vi "PolarizationSimulation.vi"() -> ()   [LabVIEW 2018]
uses:
  <vilib>/Analysis/NI_AALPro.lvlib
  <vilib>/Analysis/NI_AALBase.lvlib
panel:
  in  "STOP":bool
  in  "Microwave Power":dbl=1.0
  in  "Lower Fit\nParameter":dbl=-3.6
  in  "Upper Fit\nParameter":dbl=3.6
  in  "Std Dev Noise":dbl=0.003 step=0.0001
  out "lower x-value":dbl
  out "upper x-value":dbl
  in  "RF Control":cluster{i32, i32}(slide)={200, 230} scale=0.0..500.0
  out "p":dbl
  out "r":dbl
  in  "Saturation\nPolarization":dbl=0.8 min=0.0 max=0.99 step=0.01
  out "Reimann \nsum of Q":dbl
  out "Corrected Data (Q)":cluster{dbl[], dbl[]}(graph)
  out "Population Graphs":cluster{dbl[], "Array out":dbl[]}[](graph)
  in  "Select Target Type":u16(ring)=2 items=["H Target", "Test Case", "Deuteron"]
  in  "Reset":bool
  out "Total Polarization (P)":cluster{dbl, dbl}(graph)
  in  "Spin Manipulation\nPower Factor":dbl=0.005
  in  "Decay Spin\nManipulation":bool
  out "Reimann\nsum of P":dbl
  out "Corrected Data (P)":cluster{dbl[], dbl[]}[](graph)
  out "Signal and Fit (P)":cluster{dbl[], "Best Polynomial Fit":dbl[]}[](graph)
  in  "Positive\nPolarization":bool
  in  "Microwave on":bool
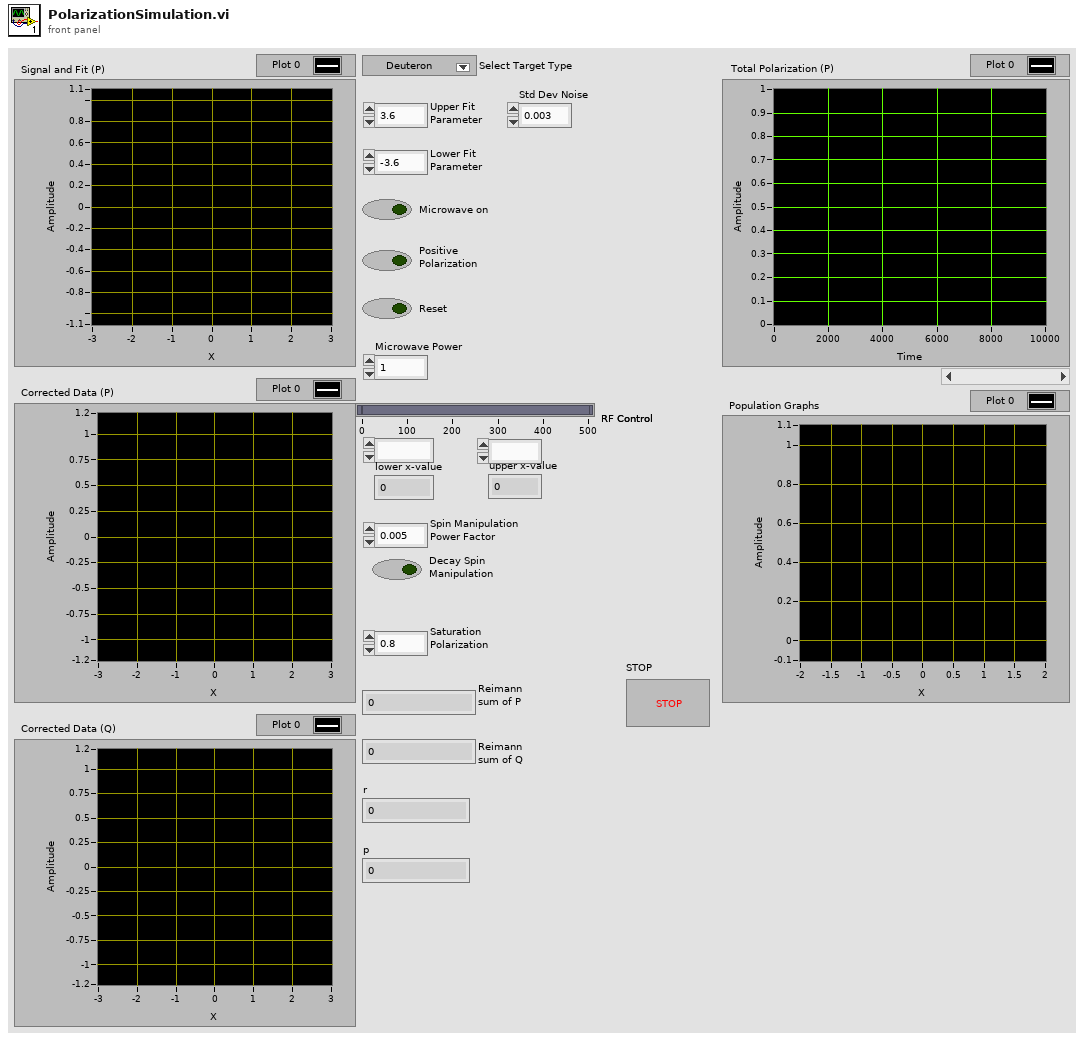
[diagram p1: front panel]
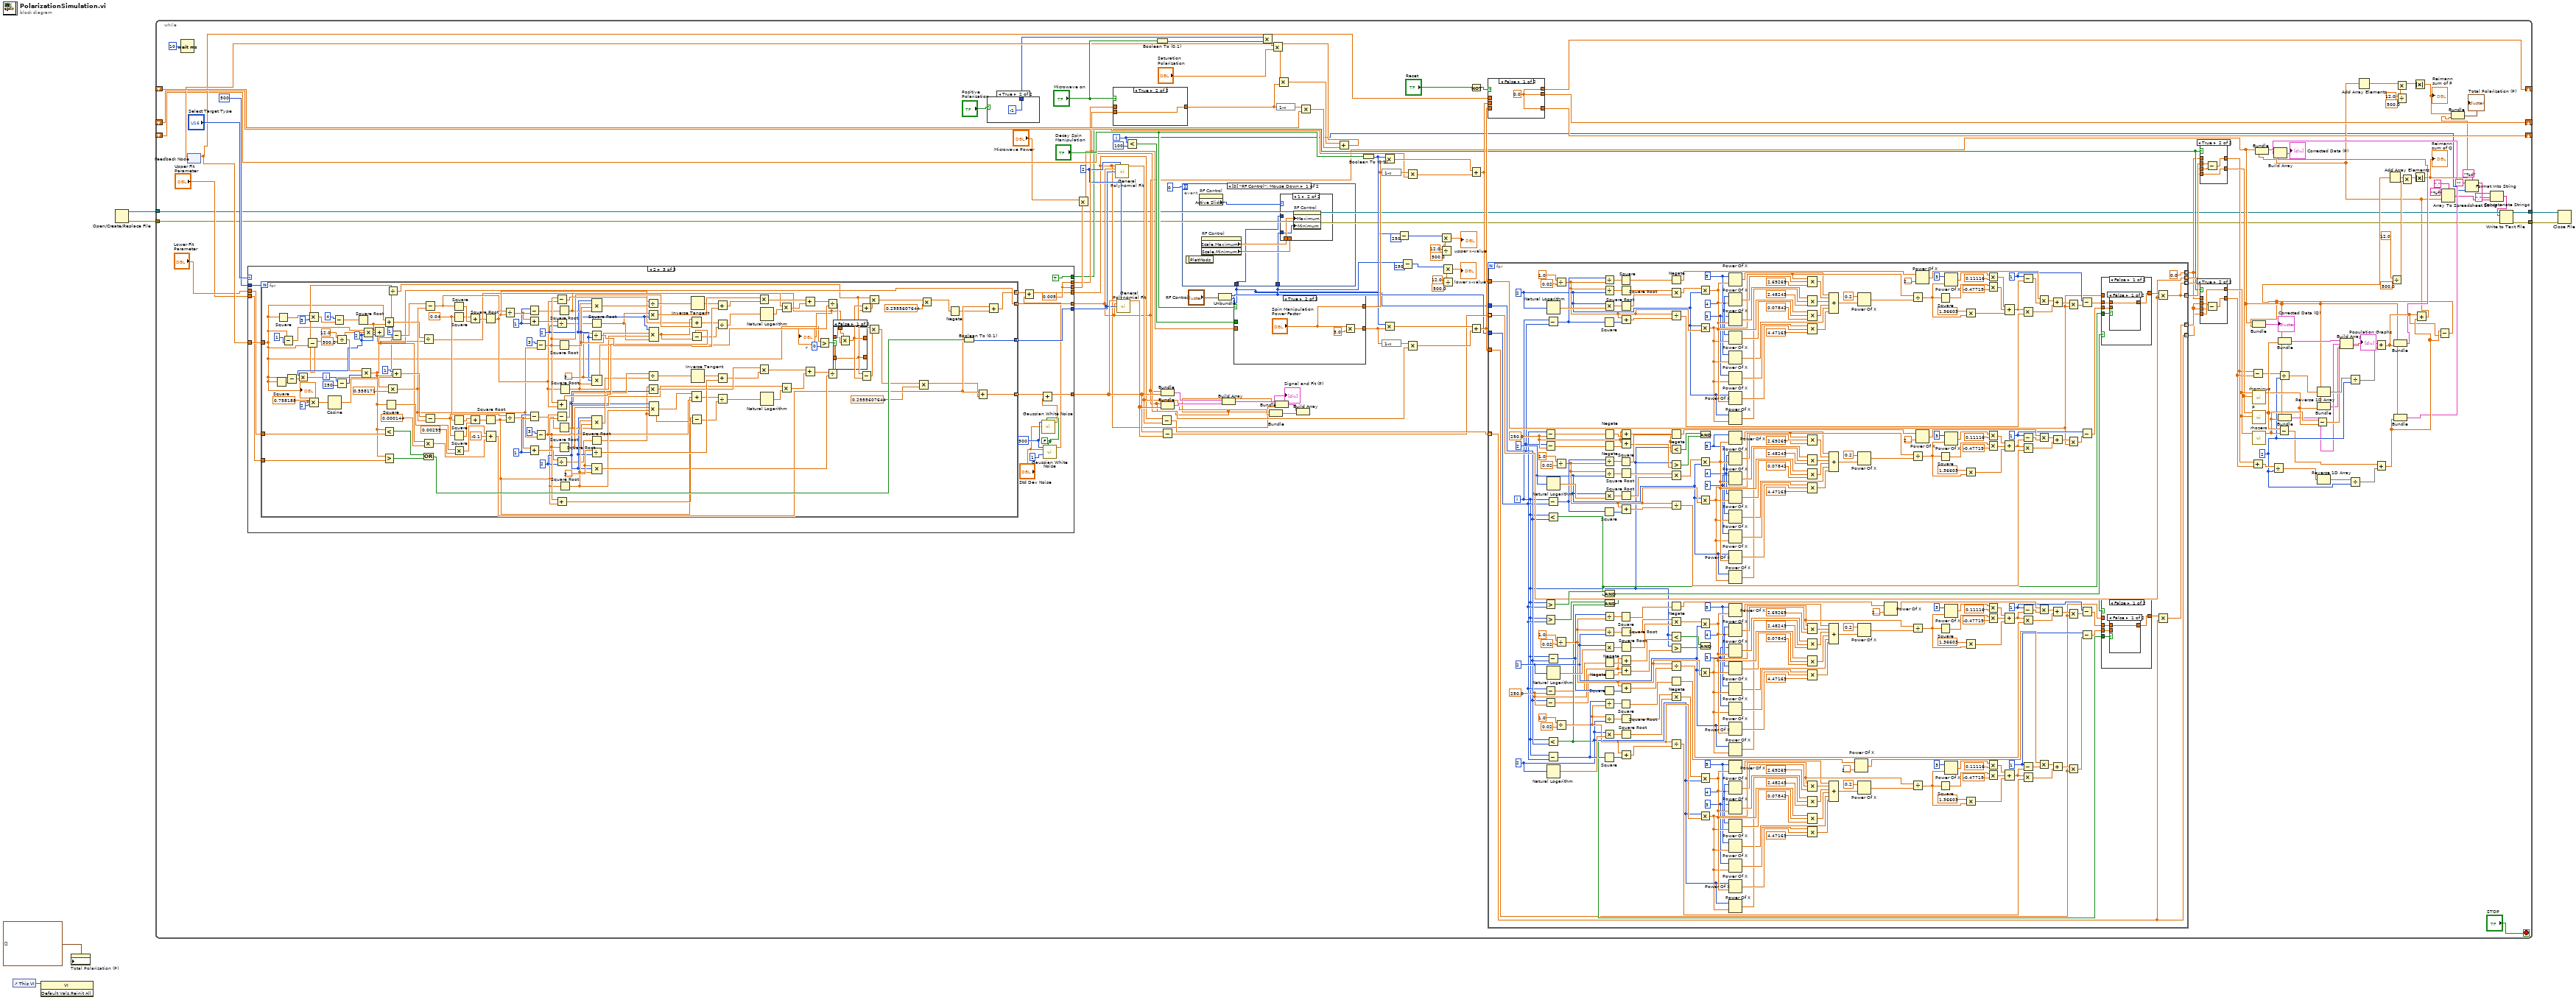
[diagram p0: block diagram]
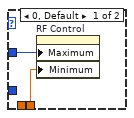
[diagram p2: hidden frame]
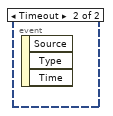
[diagram p3: hidden frame]
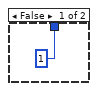
[diagram p4: hidden frame]
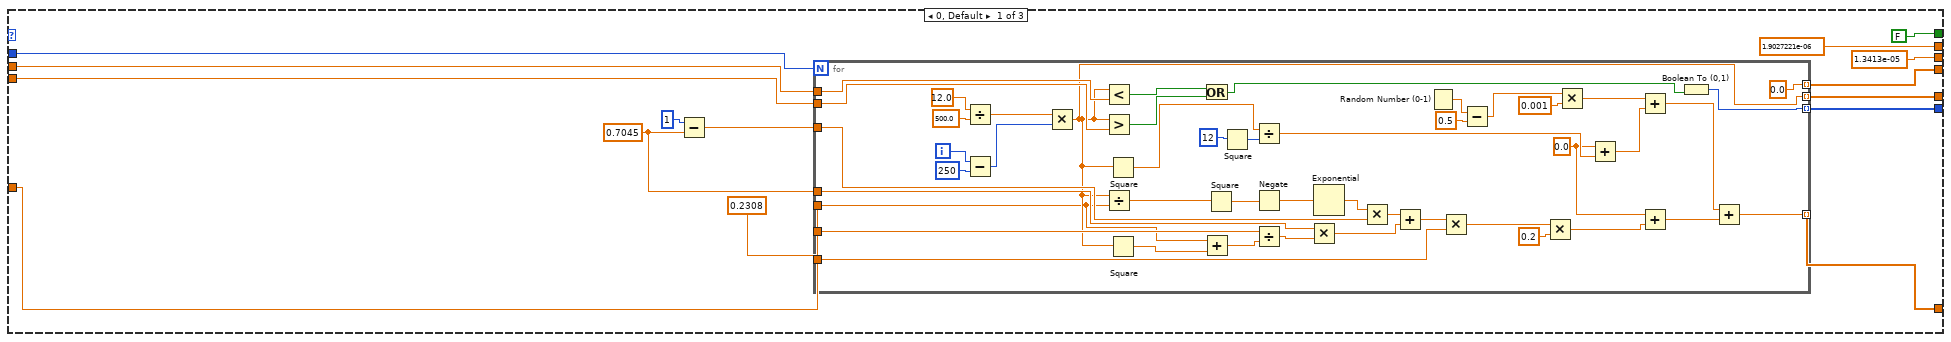
[diagram p5: hidden frame]
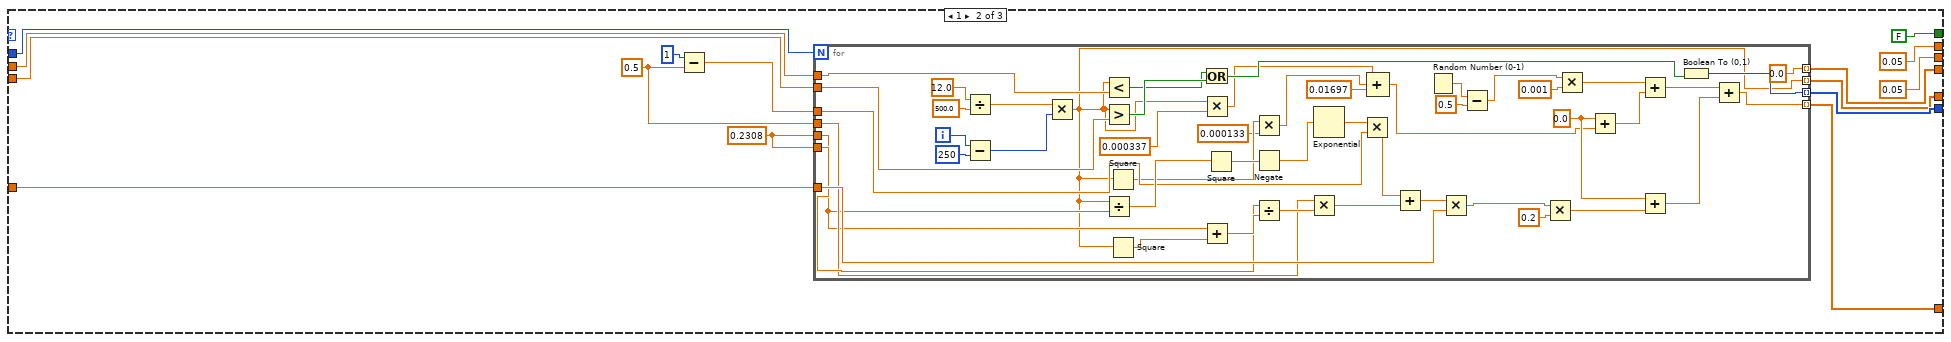
[diagram p6: hidden frame]
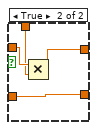
[diagram p7: hidden frame]
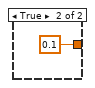
[diagram p9: hidden frame]
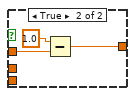
[diagram p15: hidden frame]
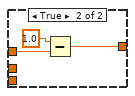
[diagram p17: hidden frame]
diagram:
  n1 = control-ref of="This VI"() -> (w6:refnum<vi>)
  n2 = invoke class="VI" method="Default Vals.Reinit All"(reference=w6) -> ()  [unwired: 2 in, 3 out]
  n3 = property on="Total Polarization (P)" class="WFChart (strict)"("History Data"=cluster{dbl, dbl}[] []) -> ()  [unwired: 2 in, 2 out]
  n4 = Open/Create/Replace File() -> (refnum out=w4:refnum<file>, error out=w3:errorcluster)  [unwired: 6 in, 1 out]
  n5 = while {
    shift-right: [w130] -> _
    shift-left: _ -> [w137]
    shift-right: [w129] -> _
    shift-left: _ -> [w109]
    shift-right: [w104] -> _
    shift-left: _ -> [w103]
    tunnel: w4 -> [w21]
    tunnel: w3 -> [w20]
    tunnel: [w19] -> w2
    tunnel: [w18] -> w1
    i -> [w13]
    stop <- "STOP" stop-if-true
    w83 = 2
    w115 = 2
    n6 = Wait (ms)(milliseconds to wait=10) -> ()  [unwired: 1 out]
    n7 = feedback #1() -> (w113:dbl)  [unwired: 1 in]
    n8 = case shown="2" "Select Target Type" {
      tunnel: [1.3413e-05 ("Growth Constant") 0.05 ("Growth Constant") w292] -> w121
      tunnel: [1.9027221e-06 ("Decay Constant") 0.05 ("Decay Constant") w292] -> w120
      tunnel: 500 -> [w167 w228 w296]
      tunnel: w113 -> [w166 w227 w299]
      tunnel: "Upper Fit\nParameter" -> [w165 w225 w297]
      tunnel: "Lower Fit\nParameter" -> [w164 w226 w298]
      tunnel: [w160 w223 w294] -> w60
      tunnel: [w163 w222 w288] -> w118
      tunnel: [w162 w224 w295] -> w114
      tunnel: [FALSE FALSE TRUE] -> w96
      tunnel: [w157 w218 w286] -> w59
      frame 0, Default {
        w158 = 0.2308
        w159 = 0.7045
        n9 = Subtract(x=1, y=w159) -> (x-y=w169:dbl)
        n10 = for {
          N: w167 -> [_]
          tunnel: w166 -> [w215]
          tunnel: [w177] -> w160 mode=indexing
          tunnel: [w193] -> w163 mode=indexing
          tunnel: [w208] -> w162 mode=indexing
          tunnel: w169 -> [w202]
          tunnel: w158 -> [w200]
          tunnel: w158 -> [w175]
          tunnel: w159 -> [w194]
          tunnel: w165 -> [w187]
          tunnel: w164 -> [w186]
          tunnel: [0.0] -> w157 mode=indexing
          i -> [w176]
          w192 = 0.0
          n11 = Divide(x=12.0, y=500.0) -> (x/y=w178:dbl)
          n12 = Subtract(x=w176, y=250) -> (x-y=w182:i32)
          n13 = Multiply(x=w178, y=w182) -> (x*y=w177:dbl)
          n14 = Less?(x=w177, y=w186) -> (x < y?=w204:bool)
          n15 = Greater?(x=w177, y=w187) -> (0:w205:bool)
          n16 = Divide(x=w177, y=w175) -> (x/y=w216:dbl)
          n17 = Square(x=w177) -> (x^2=w214:dbl)
          n18 = Square(x=w177) -> (x^2=w199:dbl)
          n19 = Or(x=w204, y=w205) -> (x .or. y?=w206:bool)
          n20 = Add(x=w175, y=w199) -> (x+y=w201:dbl)
          n21 = Square(x=w216) -> (x^2=w217:dbl)
          n22 = Square(x=12) -> (x^2=w213:i32)
          n23 = Divide(x=w214, y=w213) -> (x/y=w203:dbl)
          n24 = Negate(x=w217) -> (-x=w189:dbl)
          n25 = Divide(x=w200, y=w201) -> (x/y=w196:dbl)
          n26 = Multiply(x=w194, y=w196) -> (x*y=w195:dbl)
          n27 = Exponential(1:w189) -> (0:w188:dbl)
          n28 = Multiply(x=w188, y=w202) -> (x*y=w198:dbl)
          n29 = Add(x=w198, y=w195) -> (x+y=w197:dbl)
          n30 = Random Number (0-1)() -> (number: 0 to 1=w185:dbl)
          n31 = Multiply(x=w197, y=w215) -> (x*y=w211:dbl)
          n32 = Subtract(x=w185, y=0.5) -> (x-y=w184:dbl)
          n33 = Multiply(x=w211, y=0.2) -> (x*y=w174:dbl)
          n34 = Multiply(x=w184, y=0.001) -> (x*y=w209:dbl)
          n35 = Add(x=w192, y=w203) -> (x+y=w191:dbl)
          n36 = Add(x=w209, y=w191) -> (x+y=w207:dbl)
          n37 = Add(x=w192, y=w174) -> (x+y=w190:dbl)
          n38 = Boolean To (0,1)(Boolean=w206) -> (0, 1=w208:i16)
          n39 = Add(x=w207, y=w190) -> (x+y=w193:dbl)
        }
      }
      frame 1 {
        w229 = 0.2308
        w230 = 0.5
        n40 = Subtract(x=1, y=w230) -> (x-y=w232:dbl)
        n41 = for {
          N: w228 -> [_]
          tunnel: w227 -> [w279]
          tunnel: [w237] -> w223 mode=indexing
          tunnel: [w261] -> w222 mode=indexing
          tunnel: [w275] -> w224 mode=indexing
          tunnel: w232 -> [w270]
          tunnel: w229 -> [w268]
          tunnel: w229 -> [w244]
          tunnel: w230 -> [w262]
          tunnel: w225 -> [w255]
          tunnel: w226 -> [w254]
          tunnel: [0.0] -> w218 mode=indexing
          i -> [w245]
          w260 = 0.0
          n42 = Divide(x=12.0, y=500.0) -> (x/y=w246:dbl)
          n43 = Subtract(x=w245, y=250) -> (x-y=w250:i32)
          n44 = Multiply(x=w246, y=w250) -> (x*y=w237:dbl)
          n45 = Less?(x=w237, y=w254) -> (x < y?=w271:bool)
          n46 = Greater?(x=w237, y=w255) -> (0:w272:bool)
          n47 = Divide(x=w237, y=w244) -> (x/y=w280:dbl)
          n48 = Square(x=w237) -> (x^2=w240:dbl)
          n49 = Square(x=w237) -> (x^2=w267:dbl)
          n50 = Or(x=w271, y=w272) -> (x .or. y?=w273:bool)
          n51 = Multiply(x=w237, y=0.000337) -> (x*y=w239:dbl)
          n52 = Add(x=w244, y=w267) -> (x+y=w269:dbl)
          n53 = Square(x=w280) -> (x^2=w281:dbl)
          n54 = Multiply(x=w240, y=0.000133) -> (x*y=w238:dbl)
          n55 = Negate(x=w281) -> (-x=w257:dbl)
          n56 = Divide(x=w268, y=w269) -> (x/y=w264:dbl)
          n57 = Multiply(x=w262, y=w264) -> (x*y=w263:dbl)
          n58 = Exponential(1:w257) -> (0:w256:dbl)
          n59 = Multiply(x=w256, y=w270) -> (x*y=w266:dbl)
          n60 = Compound Arithmetic op=ADD(w239, w238, 0.01697) -> (w241:dbl)
          n61 = Add(x=w266, y=w263) -> (x+y=w265:dbl)
          n62 = Random Number (0-1)() -> (number: 0 to 1=w253:dbl)
          n63 = Multiply(x=w265, y=w279) -> (x*y=w278:dbl)
          n64 = Subtract(x=w253, y=0.5) -> (x-y=w252:dbl)
          n65 = Multiply(x=w278, y=0.2) -> (x*y=w243:dbl)
          n66 = Multiply(x=w252, y=0.001) -> (x*y=w276:dbl)
          n67 = Add(x=w260, y=w241) -> (x+y=w259:dbl)
          n68 = Add(x=w276, y=w259) -> (x+y=w274:dbl)
          n69 = Add(x=w260, y=w243) -> (x+y=w258:dbl)
          n70 = Boolean To (0,1)(Boolean=w273) -> (0, 1=w275:i16)
          n71 = Add(x=w274, y=w258) -> (x+y=w261:dbl)
        }
      }
      frame 2 {
        w283 = FALSE
        w289 = 500
        w292 = 0.005
        n72 = for {
          N: w296 -> [_]
          tunnel: [w332] -> w294 mode=indexing
          tunnel: [w421] -> w295 mode=indexing
          tunnel: w297 -> [w420]
          tunnel: w298 -> [w419]
          tunnel: [w323] -> w293 mode=indexing
          tunnel: w299 -> [w300]
          tunnel: [w324] -> w290 mode=indexing
          i -> [w397]
          w315 = 2
          w358 = 1
          w362 = 3.141592653589793
          w356 = 2
          w341 = 0.04
          w394 = 1
          w399 = 3.141592653589793
          w392 = 2
          n73 = Square(x=w300) -> (x^2=w318:dbl)
          n74 = Square(x=w300) -> (x^2=w348:dbl)
          n75 = Subtract(x=w300, y=1) -> (x-y=w343:dbl)
          n76 = Subtract(x=w300, y=w318) -> (x-y=w317:dbl)
          n77 = Multiply(x=w315, y=w317) -> (x*y=w313:dbl)
          n78 = Multiply(x=w348, y=3) -> (x*y=w347:dbl)
          n79 = Multiply(x=0.758188, y=2) -> (x*y=w336:dbl)
          n80 = Cosine(x=w336) -> (cos(x)=w339:dbl)
          n81 = Subtract(x=4, y=w347) -> (x-y=w345:dbl)
          n82 = Divide(x=12.0, y=500.0) -> (x/y=w435:dbl)
          n83 = Subtract(x=w397, y=250) -> (x-y=w434:i32)
          n84 = Square Root(x=w345) -> (sqrt(x)=w316:dbl)
          n85 = Multiply(x=w435, y=w434) -> (x*y=w332:dbl)
          n86 = Multiply(x=w343, y=w315) -> (x*y=w327:dbl)
          n87 = Add(x=w316, y=w315) -> (x+y=w314:dbl)
          n88 = Subtract(x=w314, y=w300) -> (x-y=w312:dbl)
          n89 = Add(x=w300, y=w316) -> (x+y=w344:dbl)
          n90 = Less?(x=w332, y=w419) -> (x < y?=w424:bool)
          n91 = Greater?(x=w332, y=w420) -> (0:w423:bool)
          n92 = Square(x=w332) -> (x^2=w334:dbl)
          n93 = Multiply(x=w339, y=0.558171) -> (x*y=w340:dbl)
          n94 = Divide(x=w313, y=w312) -> (x/y=w311:dbl)
          n95 = Subtract(x=1, y=w332) -> (x-y=w429:dbl)
          n96 = Add(x=1, y=w332) -> (x+y=w386:dbl)
          n97 = Divide(x=w344, y=w327) -> (x/y=w319:dbl)
          "r" <- w319
          n98 = Multiply(x=w332, y=0.000144) -> (x*y=w329:dbl)
          n99 = Or(x=w424, y=w423) -> (x .or. y?=w422:bool)
          n100 = Subtract(x=w429, y=w340) -> (x-y=w425:dbl)
          n101 = Subtract(x=w386, y=w340) -> (x-y=w382:dbl)
          n102 = Square(x=w425) -> (x^2=w428:dbl)
          n103 = Square(x=w341) -> (x^2=w427:dbl)
          n104 = Square(x=w341) -> (x^2=w384:dbl)
          n105 = Square(x=w382) -> (x^2=w385:dbl)
          n106 = Multiply(x=w334, y=0.00295) -> (x*y=w333:dbl)
          n107 = Add(x=w427, y=w428) -> (x+y=w426:dbl)
          n108 = Add(x=w384, y=w385) -> (x+y=w383:dbl)
          n109 = Square Root(x=w426) -> (sqrt(x)=w389:dbl)
          n110 = Square Root(x=w383) -> (sqrt(x)=w353:dbl)
          n111 = Compound Arithmetic op=ADD(w333, -0.1, w329) -> (w325:dbl)
          n112 = Divide(x=w425, y=w389) -> (x/y=w395:dbl)
          n113 = Divide(x=w382, y=w353) -> (x/y=w359:dbl)
          n114 = Subtract(x=w394, y=w395) -> (x-y=w350:dbl)
          n115 = Add(x=w395, y=w394) -> (x+y=w393:dbl)
          n116 = Subtract(x=w358, y=w359) -> (x-y=w351:dbl)
          n117 = Add(x=w359, y=w358) -> (x+y=w357:dbl)
          n118 = Subtract(x=3, y=w340) -> (x-y=w405:dbl)
          n119 = Subtract(x=3, y=w340) -> (x-y=w368:dbl)
          n120 = Subtract(x=w405, y=w389) -> (x-y=w414:dbl)
          n121 = Divide(x=w393, y=w392) -> (x/y=w391:dbl)
          n122 = Add(x=w405, y=w389) -> (x+y=w404:dbl)
          n123 = Subtract(x=w368, y=w353) -> (x-y=w377:dbl)
          n124 = Divide(x=w357, y=w356) -> (x/y=w355:dbl)
          n125 = Add(x=w368, y=w353) -> (x+y=w367:dbl)
          n126 = Square Root(x=w350) -> (sqrt(x)=w396:dbl)
          n127 = Square Root(x=w405) -> (sqrt(x)=w408:dbl)
          n128 = Square Root(x=w351) -> (sqrt(x)=w360:dbl)
          n129 = Square Root(x=w368) -> (sqrt(x)=w371:dbl)
          n130 = Square Root(x=w389) -> (sqrt(x)=w398:dbl)
          n131 = Square Root(x=w353) -> (sqrt(x)=w361:dbl)
          n132 = Square Root(x=w391) -> (sqrt(x)=w390:dbl)
          n133 = Divide(x=w399, y=w392) -> (x/y=w416:dbl)
          n134 = Square Root(x=w355) -> (sqrt(x)=w354:dbl)
          n135 = Divide(x=w362, y=w356) -> (x/y=w379:dbl)
          n136 = Compound Arithmetic op=MULTIPLY(w392, w398, w408, w396) -> (w413:dbl)
          n137 = Compound Arithmetic op=MULTIPLY(w399, w392, w398) -> (w400:dbl)
          n138 = Compound Arithmetic op=MULTIPLY(w356, w361, w371, w360) -> (w376:dbl)
          n139 = Compound Arithmetic op=MULTIPLY(w362, w356, w361) -> (w363:dbl)
          n140 = Divide(x=w414, y=w413) -> (x/y=w412:dbl)
          n141 = Multiply(x=w390, y=w392) -> (x*y=w418:dbl)
          n142 = Divide(x=w377, y=w376) -> (x/y=w375:dbl)
          n143 = Multiply(x=w354, y=w356) -> (x*y=w381:dbl)
          n144 = Compound Arithmetic op=MULTIPLY(w392, w408, w398, w390) -> (w403:dbl)
          n145 = Compound Arithmetic op=MULTIPLY(w356, w371, w361, w354) -> (w366:dbl)
          n146 = Subtract(x=w404, y=w403) -> (x-y=w402:dbl)
          n147 = Subtract(x=w367, y=w366) -> (x-y=w365:dbl)
          n148 = Inverse Tangent(1:w412) -> (0:w417:dbl)
          n149 = Inverse Tangent(1:w375) -> (0:w380:dbl)
          n150 = Compound Arithmetic op=ADD(w403, w389, w405) -> (w407:dbl)
          n151 = Compound Arithmetic op=ADD(w366, w353, w368) -> (w370:dbl)
          n152 = Add(x=w417, y=w416) -> (x+y=w415:dbl)
          n153 = Divide(x=w407, y=w402) -> (x/y=w406:dbl)
          n154 = Add(x=w380, y=w379) -> (x+y=w378:dbl)
          n155 = Divide(x=w370, y=w365) -> (x/y=w369:dbl)
          n156 = Multiply(x=w418, y=w415) -> (x*y=w411:dbl)
          n157 = Multiply(x=w381, y=w378) -> (x*y=w374:dbl)
          n158 = Natural Logarithm(1:w406) -> (0:w409:dbl)
          n159 = Natural Logarithm(1:w369) -> (0:w372:dbl)
          n160 = Multiply(x=w396, y=w409) -> (x*y=w410:dbl)
          n161 = Multiply(x=w360, y=w372) -> (x*y=w373:dbl)
          n162 = Add(x=w411, y=w410) -> (x+y=w401:dbl)
          n163 = Add(x=w374, y=w373) -> (x+y=w364:dbl)
          n164 = Greater?(x=w300, y=0) -> (0:w302:bool)
          n165 = Divide(x=w401, y=w400) -> (x/y=w342:dbl)
          n166 = Divide(x=w364, y=w363) -> (x/y=w304:dbl)
          n167 = case shown="False" w302 {
            tunnel: w342 -> [w439 w444]
            tunnel: [w437 w443] -> w322
            tunnel: w319 -> [w440 w442]
            tunnel: w304 -> [w438 w441]
            tunnel: [w438 w441] -> w303
            frame False {
              n168 = Multiply(x=w440, y=w439) -> (x*y=w437:dbl)
            }
            frame True {
              n169 = Multiply(x=w444, y=w442) -> (x*y=w443:dbl)
            }
          }
          n170 = Add(x=w322, y=w303) -> (x+y=w326:dbl)
          n171 = Subtract(x=w303, y=w322) -> (x-y=w352:dbl)
          n172 = Multiply(x=w311, y=w326) -> (x*y=w310:dbl)
          n173 = Multiply(x=w311, y=w352) -> (x*y=w309:dbl)
          n174 = Multiply(x=w309, y=0.2955607644) -> (x*y=w306:dbl)
          n175 = Multiply(x=w310, y=0.2955607644) -> (x*y=w308:dbl)
          n176 = Negate(x=w308) -> (-x=w321:dbl)
          n177 = Boolean To (0,1)(Boolean=w422) -> (0, 1=w421:i16)
          n178 = Add(x=w325, y=w306) -> (x+y=w323:dbl)
          n179 = Add(x=w325, y=w321) -> (x+y=w324:dbl)
          "p" <- w300
        }
        n180 = call <vilib>:"Gaussian White Noise.vi"("initialize?"=w283, "standard deviation"="Std Dev Noise", "samples"=w289) -> ("Gaussian noise pattern"=w287:dbl[])  [unwired: 7 in, 1 out]
        n181 = Add(x=w293, y=w287) -> (x+y=w288:dbl[])
        n182 = call <vilib>:"Gaussian White Noise.vi"("initialize?"=w283, "seed"=1, "standard deviation"="Std Dev Noise", "samples"=w289) -> ("Gaussian noise pattern"=w285:dbl[])  [unwired: 6 in, 1 out]
        n183 = Add(x=w290, y=w285) -> (x+y=w286:dbl[])
      }
    }
    n184 = case shown="True" "Positive\nPolarization" {
      tunnel: [1 -1] -> w56
      frame False {
      }
      frame True {
      }
    }
    n185 = Multiply(x="Microwave Power", y=w121) -> (x*y=w24:dbl)
    n186 = case shown="True" "Microwave on" {
      tunnel: [w453 w454] -> w124
      tunnel: w24 -> [_ w454]
      tunnel: w120 -> [w453 _]
      frame False {
      }
      frame True {
      }
    }
    n187 = call <vilib>:"General Polynomial Fit.vi"("Y"=w59, "polynomial order"=w115, "X"=w60, "Weight"=w114) -> ("Best Polynomial Fit"=w62:dbl[])  [unwired: 8 in, 3 out]
    n188 = call <vilib>:"General Polynomial Fit.vi"("Y"=w118, "polynomial order"=w115, "X"=w60, "Weight"=w114) -> ("Best Polynomial Fit"=w143:dbl[])  [unwired: 8 in, 3 out]
    n189 = Less?(x=w13, y=100) -> (x < y?=w132:bool)
    n190 = Boolean To (0,1)(Boolean="Microwave on") -> (0, 1=w139:i16)
    n191 = Subtract(x=w59, y=w62) -> (x-y=w76:dbl[])
    n192 = Bundle(w60, w118) -> (w144:cluster{dbl[], dbl[]})  [unwired: 1 in]
    n193 = Bundle(w60, "Best Polynomial Fit"=w143) -> (w64:cluster{dbl[], "Best Polynomial Fit":dbl[]})  [unwired: 1 in]
    n194 = Subtract(x=w118, y=w143) -> (x-y=w75:dbl[])
    n195 = Unbundle("RF Control") -> (w27:i32, w26:i32)
    n196 = event shown="[0] \"RF Control\": Mouse Down" {
      selector: _ -> [_ _]
      dyn-events: _ -> [_ _]
      timeout: 0 -> [_ _]
      tunnel: w27 -> [w147 _]
      tunnel: w26 -> [w146 _]
      event "RF Control": Mouse Down {
        n197 = event-data() -> ()  [unwired: 1 in, 1 out]
        n198 = property on="RF Control" class="Slide (strict)"() -> ("Active Slider"=w150:i32)  [unwired: 2 in, 2 out]
        n199 = property on="RF Control" class="Slide (strict)"() -> ("Scale.Maximum"=w148:dbl, "Scale.Minimum"=w149:dbl)  [unwired: 2 in, 2 out]
        n200 = case shown="1" w150 {
          tunnel: w149 -> [w152 _]
          tunnel: w146 -> [w151 _]
          tunnel: w148 -> [_ w154]
          tunnel: w147 -> [_ w153]
          frame 0, Default {
            n201 = property on="RF Control" class="Slide (strict)"("Maximum"=w151, "Minimum"=w152) -> ()  [unwired: 2 in, 2 out]
          }
          frame 1 {
            n202 = property on="RF Control" class="Slide (strict)"("Maximum"=w154, "Minimum"=w153) -> ()  [unwired: 2 in, 2 out]
          }
        }
      }
      event Timeout {
        n203 = event-data() -> ()  [unwired: 1 in, 3 out]
      }
    }
    n204 = Build Array(w144, w64) -> (→"Signal and Fit (P)":cluster{dbl[], "Best Polynomial Fit":dbl[]}[])
    n205 = case shown="True" "Decay Spin\nManipulation" {
      tunnel: [w445 "Spin Manipulation\nPower Factor"] -> w133
      tunnel: w24 -> [w447 _]
      tunnel: w132 -> [w446 _]
      tunnel: [w445 w450] -> w111
      frame False {
        n206 = case shown="False" w446 {
          tunnel: [w448 0.1] -> w445
          tunnel: w447 -> [w448 _]
          frame False {
          }
          frame True {
          }
        }
      }
      frame True {
        n207 = Multiply(x="Spin Manipulation\nPower Factor", y=3.0) -> (x*y=w450:dbl)
      }
    }
    n208 = Multiply(x=w56, y=w139) -> (x*y=w57:i32)
    n209 = Bundle(w60, "Best Polynomial Fit"=w62) -> (w63:cluster{dbl[], "Best Polynomial Fit":dbl[]})  [unwired: 1 in]
    n210 = Multiply(x=w57, y="Saturation\nPolarization") -> (x*y=w74:dbl)
    n211 = Bundle(w60, w59) -> (w61:cluster{dbl[], dbl[]})  [unwired: 1 in]
    n212 = expression code="1-x"(w124) -> (w140:dbl)
    n213 = Multiply(x=w74, y=w124) -> (x*y=w141:dbl)
    n214 = Build Array(w61, w63) -> ()  [unwired: 1 out]
    n215 = Multiply(x=w140, y=w137) -> (x*y=w142:dbl)
    n216 = Add(x=w141, y=w142) -> (x+y=w119:dbl)
    n217 = feedback-in #1(w119) -> ()
    n218 = Boolean To (0,1)(Boolean="Decay Spin\nManipulation") -> (0, 1=w112:i16)
    n219 = expression code="1-x"(w133) -> (w134:dbl)
    n220 = expression code="1-x"(w111) -> (w110:dbl)
    n221 = Multiply(x=w112, y=w133) -> (x*y=w135:dbl)
    n222 = Multiply(x=w112, y=w111) -> (x*y=w107:dbl)
    n223 = Subtract(x=w26, y=250) -> (x-y=w36:i32)
    n224 = Subtract(x=w27, y=250) -> (x-y=w33:i32)
    n225 = Multiply(x=w134, y=w109) -> (x*y=w136:dbl)
    n226 = Multiply(x=w110, y=w103) -> (x*y=w108:dbl)
    n227 = Divide(x=12.0, y=500.0) -> (x/y=w44:dbl)
    n228 = Multiply(x=w36, y=w44) -> (x*y=→"upper x-value":dbl)
    n229 = Divide(x=12.0, y=500.0) -> (x/y=w40:dbl)
    n230 = Multiply(x=w33, y=w40) -> (x*y=→"lower x-value":dbl)
    n231 = Not(x="Reset") -> (.not. x?=w127:bool)
    n232 = Add(x=w135, y=w136) -> (x+y=w128:dbl)
    n233 = Add(x=w107, y=w108) -> (x+y=w105:dbl)
    n234 = case shown="False" w127 {
      tunnel: [w467 w470] -> w130
      tunnel: w113 -> [_ w470]
      tunnel: [w467 w469] -> w129
      tunnel: w128 -> [_ w469]
      tunnel: w105 -> [_ w468]
      tunnel: [w467 w468] -> w104
      frame False {
        w467 = 0.0
      }
      frame True {
      }
    }
    n235 = for {
      tunnel: w75 -> [w614] mode=indexing
      tunnel: w128 -> [w622]
      tunnel: w26 -> [w478]
      tunnel: w27 -> [w477]
      tunnel: [w614] -> w117 mode=indexing
      tunnel: [w613] -> w106 mode=indexing
      tunnel: [w613] -> w116 mode=indexing
      tunnel: w76 -> [w472] mode=indexing
      tunnel: w105 -> [w476]
      tunnel: [w474] -> w101 mode=indexing
      tunnel: [w472] -> w100 mode=indexing
      tunnel: [0.0] -> w90 mode=indexing
      i -> [w475]
      w480 = 250.0
      w519 = 5
      w517 = 4
      w516 = 3
      w497 = 1
      w498 = 2
      w580 = 5
      w578 = 4
      w577 = 3
      w557 = 1
      w558 = 2
      w616 = 250.0
      w657 = 5
      w655 = 4
      w654 = 3
      w635 = 1
      w636 = 2
      w718 = 5
      w716 = 4
      w715 = 3
      w695 = 1
      w696 = 2
      n236 = Subtract(x=w477, y=w616) -> (x-y=w620:dbl)
      n237 = Subtract(x=w478, y=w616) -> (x-y=w621:dbl)
      n238 = Greater?(x=w475, y=w477) -> (0:w691:bool)
      n239 = Greater?(x=w475, y=w477) -> (0:w553:bool)
      n240 = Subtract(x=w477, y=w480) -> (x-y=w484:dbl)
      n241 = Subtract(x=w478, y=w480) -> (x-y=w485:dbl)
      n242 = Natural Logarithm(1:w636) -> (0:w670:dbl)
      n243 = Subtract(x=w475, y=w478) -> (x-y=w643:i32)
      n244 = Natural Logarithm(1:w696) -> (0:w731:dbl)
      n245 = Subtract(x=w475, y=w477) -> (x-y=w704:i32)
      n246 = Less?(x=w475, y=w478) -> (x < y?=w627:bool)
      n247 = Subtract(x=w475, y=w478) -> (x-y=w505:i32)
      n248 = Natural Logarithm(1:w498) -> (0:w532:dbl)
      n249 = Less?(x=w475, y=w478) -> (x < y?=w490:bool)
      n250 = Subtract(x=w475, y=w477) -> (x-y=w566:i32)
      n251 = Natural Logarithm(1:w558) -> (0:w593:dbl)
      n252 = Divide(x=1.0, y=0.02) -> (x/y=w640:dbl)
      n253 = Divide(x=1.0, y=0.02) -> (x/y=w700:dbl)
      n254 = Divide(x=1.0, y=0.02) -> (x/y=w502:dbl)
      n255 = Divide(x=1.0, y=0.02) -> (x/y=w562:dbl)
      n256 = Square(x=w643) -> (x^2=w644:i32)
      n257 = Square(x=w704) -> (x^2=w705:i32)
      n258 = Square(x=w505) -> (x^2=w506:i32)
      n259 = Square(x=w566) -> (x^2=w567:i32)
      n260 = Divide(x=w643, y=w640) -> (x/y=w647:dbl)
      n261 = Divide(x=w640, y=w636) -> (x/y=w668:dbl)
      n262 = Multiply(x=w636, y=w670) -> (x*y=w671:dbl)
      n263 = Negate(x=w620) -> (-x=w619:dbl)
      n264 = Negate(x=w621) -> (-x=w617:dbl)
      n265 = Divide(x=w704, y=w700) -> (x/y=w708:dbl)
      n266 = Divide(x=w700, y=w696) -> (x/y=w729:dbl)
      n267 = Multiply(x=w696, y=w731) -> (x*y=w732:dbl)
      n268 = Divide(x=w505, y=w502) -> (x/y=w509:dbl)
      n269 = Divide(x=w502, y=w498) -> (x/y=w530:dbl)
      n270 = Multiply(x=w498, y=w532) -> (x*y=w533:dbl)
      n271 = Negate(x=w484) -> (-x=w483:dbl)
      n272 = Negate(x=w485) -> (-x=w481:dbl)
      n273 = Divide(x=w566, y=w562) -> (x/y=w570:dbl)
      n274 = Divide(x=w562, y=w558) -> (x/y=w591:dbl)
      n275 = Multiply(x=w558, y=w593) -> (x*y=w594:dbl)
      n276 = And(x=w691, y=w627) -> (x .and. y?=w629:bool)
      n277 = And(x=w553, y=w490) -> (x .and. y?=w491:bool)
      n278 = Square(x=w647) -> (x^2=w649:dbl)
      n279 = Square(x=w708) -> (x^2=w710:dbl)
      n280 = Square(x=w509) -> (x^2=w511:dbl)
      n281 = Square(x=w570) -> (x^2=w572:dbl)
      n282 = Square Root(x=w668) -> (sqrt(x)=w669:dbl)
      n283 = Square Root(x=w671) -> (sqrt(x)=w672:dbl)
      n284 = Add(x=w640, y=w644) -> (x+y=w645:dbl)
      n285 = Add(x=w616, y=w619) -> (x+y=w618:dbl)
      n286 = Add(x=w616, y=w617) -> (x+y=w615:dbl)
      n287 = Square Root(x=w729) -> (sqrt(x)=w730:dbl)
      n288 = Square Root(x=w732) -> (sqrt(x)=w733:dbl)
      n289 = Add(x=w700, y=w705) -> (x+y=w706:dbl)
      n290 = Square Root(x=w530) -> (sqrt(x)=w531:dbl)
      n291 = Square Root(x=w533) -> (sqrt(x)=w534:dbl)
      n292 = Add(x=w480, y=w483) -> (x+y=w482:dbl)
      n293 = Add(x=w480, y=w481) -> (x+y=w479:dbl)
      n294 = Add(x=w502, y=w506) -> (x+y=w507:dbl)
      n295 = Square Root(x=w591) -> (sqrt(x)=w592:dbl)
      n296 = Square Root(x=w594) -> (sqrt(x)=w595:dbl)
      n297 = Add(x=w562, y=w567) -> (x+y=w568:dbl)
      n298 = Negate(x=w649) -> (-x=w648:dbl)
      n299 = Multiply(x=w669, y=w672) -> (x*y=w663:dbl)
      n300 = Divide(x=w640, y=w645) -> (x/y=w630:dbl)
      n301 = Negate(x=w710) -> (-x=w709:dbl)
      n302 = Less?(x=w475, y=w618) -> (x < y?=w624:bool)
      n303 = Greater?(x=w475, y=w615) -> (0:w623:bool)
      n304 = Multiply(x=w730, y=w733) -> (x*y=w724:dbl)
      n305 = Divide(x=w700, y=w706) -> (x/y=w703:dbl)
      n306 = Negate(x=w511) -> (-x=w510:dbl)
      n307 = Multiply(x=w531, y=w534) -> (x*y=w525:dbl)
      n308 = Less?(x=w475, y=w482) -> (x < y?=w487:bool)
      n309 = Greater?(x=w475, y=w479) -> (0:w486:bool)
      n310 = Divide(x=w502, y=w507) -> (x/y=w492:dbl)
      n311 = Negate(x=w572) -> (-x=w571:dbl)
      n312 = Multiply(x=w592, y=w595) -> (x*y=w586:dbl)
      n313 = Divide(x=w562, y=w568) -> (x/y=w565:dbl)
      n314 = Multiply(x=w663, y=w636) -> (x*y=w687:dbl)
      n315 = Multiply(x=w636, y=w640) -> (x*y=w681:dbl)
      n316 = Multiply(x=w724, y=w696) -> (x*y=w748:dbl)
      n317 = Multiply(x=w696, y=w700) -> (x*y=w742:dbl)
      n318 = Multiply(x=w525, y=w498) -> (x*y=w549:dbl)
      n319 = Multiply(x=w498, y=w502) -> (x*y=w543:dbl)
      n320 = Multiply(x=w586, y=w558) -> (x*y=w610:dbl)
      n321 = Multiply(x=w558, y=w562) -> (x*y=w604:dbl)
      n322 = And(x=w624, y=w623) -> ()  [unwired: 1 out]
      n323 = And(x=w487, y=w486) -> ()  [unwired: 1 out]
      n324 = Power Of X(1:w687, 2:w657) -> (0:w674:dbl)
      n325 = Power Of X(1:w687, 2:w655) -> (0:w680:dbl)
      n326 = Power Of X(1:w687, 2:w654) -> (0:w682:dbl)
      n327 = Power Of X(1:w681, 2:w655) -> (0:w686:dbl)
      n328 = Power Of X(1:w681, 2:w657) -> (0:w675:dbl)
      n329 = Power Of X(1:w681, 2:w654) -> (0:w684:dbl)
      n330 = Power Of X(1:w687, 2:w636) -> (0:w685:dbl)
      n331 = Power Of X(1:w681, 2:w636) -> (0:w683:dbl)
      n332 = Power Of X(1:w748, 2:w718) -> (0:w735:dbl)
      n333 = Power Of X(1:w748, 2:w716) -> (0:w741:dbl)
      n334 = Power Of X(1:w748, 2:w715) -> (0:w743:dbl)
      n335 = Power Of X(1:w742, 2:w716) -> (0:w747:dbl)
      n336 = Power Of X(1:w742, 2:w718) -> (0:w736:dbl)
      n337 = Power Of X(1:w742, 2:w715) -> (0:w745:dbl)
      n338 = Power Of X(1:w748, 2:w696) -> (0:w746:dbl)
      n339 = Power Of X(1:w742, 2:w696) -> (0:w744:dbl)
      n340 = Power Of X(1:w549, 2:w519) -> (0:w536:dbl)
      n341 = Power Of X(1:w549, 2:w517) -> (0:w542:dbl)
      n342 = Power Of X(1:w549, 2:w516) -> (0:w544:dbl)
      n343 = Power Of X(1:w543, 2:w517) -> (0:w548:dbl)
      n344 = Power Of X(1:w543, 2:w519) -> (0:w537:dbl)
      n345 = Power Of X(1:w543, 2:w516) -> (0:w546:dbl)
      n346 = Power Of X(1:w549, 2:w498) -> (0:w547:dbl)
      n347 = Power Of X(1:w543, 2:w498) -> (0:w545:dbl)
      n348 = Power Of X(1:w610, 2:w580) -> (0:w597:dbl)
      n349 = Power Of X(1:w610, 2:w578) -> (0:w603:dbl)
      n350 = Power Of X(1:w610, 2:w577) -> (0:w605:dbl)
      n351 = Power Of X(1:w604, 2:w578) -> (0:w609:dbl)
      n352 = Power Of X(1:w604, 2:w580) -> (0:w598:dbl)
      n353 = Power Of X(1:w604, 2:w577) -> (0:w607:dbl)
      n354 = Power Of X(1:w610, 2:w558) -> (0:w608:dbl)
      n355 = Power Of X(1:w604, 2:w558) -> (0:w606:dbl)
      n356 = Compound Arithmetic op=MULTIPLY(w681, w680, 2.69269) -> (w676:dbl)
      n357 = Compound Arithmetic op=MULTIPLY(w682, w683, 2.48243) -> (w678:dbl)
      n358 = Compound Arithmetic op=MULTIPLY(w687, w686, 0.07842) -> (w677:dbl)
      n359 = Compound Arithmetic op=MULTIPLY(w684, w685, 4.47163) -> (w679:dbl)
      n360 = Compound Arithmetic op=MULTIPLY(w742, w741, 2.69269) -> (w737:dbl)
      n361 = Compound Arithmetic op=MULTIPLY(w743, w744, 2.48243) -> (w739:dbl)
      n362 = Compound Arithmetic op=MULTIPLY(w748, w747, 0.07842) -> (w738:dbl)
      n363 = Compound Arithmetic op=MULTIPLY(w745, w746, 4.47163) -> (w740:dbl)
      n364 = Compound Arithmetic op=MULTIPLY(w543, w542, 2.69269) -> (w538:dbl)
      n365 = Compound Arithmetic op=MULTIPLY(w544, w545, 2.48243) -> (w540:dbl)
      n366 = Compound Arithmetic op=MULTIPLY(w549, w548, 0.07842) -> (w539:dbl)
      n367 = Compound Arithmetic op=MULTIPLY(w546, w547, 4.47163) -> (w541:dbl)
      n368 = Compound Arithmetic op=MULTIPLY(w604, w603, 2.69269) -> (w599:dbl)
      n369 = Compound Arithmetic op=MULTIPLY(w605, w606, 2.48243) -> (w601:dbl)
      n370 = Compound Arithmetic op=MULTIPLY(w610, w609, 0.07842) -> (w600:dbl)
      n371 = Compound Arithmetic op=MULTIPLY(w607, w608, 4.47163) -> (w602:dbl)
      n372 = Compound Arithmetic op=unknown(w674, w676, w678, w677, w675, w679) -> (w637:dbl)
      n373 = Compound Arithmetic op=unknown(w735, w737, w739, w738, w736, w740) -> (w697:dbl)
      n374 = Compound Arithmetic op=unknown(w536, w538, w540, w539, w537, w541) -> (w499:dbl)
      n375 = Compound Arithmetic op=unknown(w597, w599, w601, w600, w598, w602) -> (w559:dbl)
      n376 = Power Of X(1:2.718281828459045, 2:w571) -> (0:w569:dbl)
      n377 = Power Of X(1:w637, 2:0.2) -> (0:w689:dbl)
      n378 = Power Of X(1:w697, 2:0.2) -> (0:w750:dbl)
      n379 = Power Of X(1:w499, 2:0.2) -> (0:w551:dbl)
      n380 = Power Of X(1:w559, 2:0.2) -> (0:w612:dbl)
      n381 = Power Of X(1:2.718281828459045, 2:w510) -> (0:w508:dbl)
      n382 = Divide(x=w681, y=w689) -> (x/y=w673:dbl)
      n383 = Divide(x=w742, y=w750) -> (x/y=w734:dbl)
      n384 = Divide(x=w543, y=w551) -> (x/y=w535:dbl)
      n385 = Divide(x=w604, y=w612) -> (x/y=w596:dbl)
      n386 = Power Of X(1:2.718281828459045, 2:w648) -> (0:w646:dbl)
      n387 = Power Of X(1:2.718281828459045, 2:w709) -> (0:w707:dbl)
      n388 = Square(x=w673) -> (x^2=w667:dbl)
      n389 = Square(x=w734) -> (x^2=w728:dbl)
      n390 = Square(x=w535) -> (x^2=w529:dbl)
      n391 = Square(x=w596) -> (x^2=w590:dbl)
      n392 = Power Of X(1:w673, 2:3) -> (0:w666:dbl)
      n393 = Power Of X(1:w734, 2:3) -> (0:w727:dbl)
      n394 = Power Of X(1:w535, 2:3) -> (0:w528:dbl)
      n395 = Power Of X(1:w596, 2:3) -> (0:w589:dbl)
      n396 = Multiply(x=1.36603, y=w673) -> (x*y=w688:dbl)
      n397 = Multiply(x=1.36603, y=w734) -> (x*y=w749:dbl)
      n398 = Multiply(x=1.36603, y=w535) -> (x*y=w550:dbl)
      n399 = Multiply(x=1.36603, y=w596) -> (x*y=w611:dbl)
      n400 = Multiply(x=w666, y=0.11116) -> (x*y=w665:dbl)
      n401 = Multiply(x=w667, y=-0.47719) -> (x*y=w664:dbl)
      n402 = Multiply(x=w727, y=0.11116) -> (x*y=w726:dbl)
      n403 = Multiply(x=w728, y=-0.47719) -> (x*y=w725:dbl)
      n404 = Multiply(x=w528, y=0.11116) -> (x*y=w527:dbl)
      n405 = Multiply(x=w529, y=-0.47719) -> (x*y=w526:dbl)
      n406 = Multiply(x=w589, y=0.11116) -> (x*y=w588:dbl)
      n407 = Multiply(x=w590, y=-0.47719) -> (x*y=w587:dbl)
      n408 = Compound Arithmetic op=unknown(w665, w664, w688) -> (w641:dbl)
      n409 = Compound Arithmetic op=unknown(w726, w725, w749) -> (w701:dbl)
      n410 = Compound Arithmetic op=unknown(w527, w526, w550) -> (w503:dbl)
      n411 = Compound Arithmetic op=unknown(w588, w587, w611) -> (w563:dbl)
      n412 = Subtract(x=w635, y=w641) -> (x-y=w638:dbl)
      n413 = Multiply(x=w641, y=w630) -> (x*y=w642:dbl)
      n414 = Subtract(x=w695, y=w701) -> (x-y=w698:dbl)
      n415 = Multiply(x=w701, y=w703) -> (x*y=w702:dbl)
      n416 = Subtract(x=w497, y=w503) -> (x-y=w500:dbl)
      n417 = Multiply(x=w503, y=w492) -> (x*y=w504:dbl)
      n418 = Subtract(x=w557, y=w563) -> (x-y=w560:dbl)
      n419 = Multiply(x=w563, y=w565) -> (x*y=w564:dbl)
      n420 = Multiply(x=w646, y=w638) -> (x*y=w639:dbl)
      n421 = Multiply(x=w707, y=w698) -> (x*y=w699:dbl)
      n422 = Multiply(x=w508, y=w500) -> (x*y=w501:dbl)
      n423 = Multiply(x=w569, y=w560) -> (x*y=w561:dbl)
      n424 = Add(x=w639, y=w642) -> (x+y=w634:dbl)
      n425 = Add(x=w699, y=w702) -> (x+y=w694:dbl)
      n426 = Add(x=w501, y=w504) -> (x+y=w496:dbl)
      n427 = Add(x=w561, y=w564) -> (x+y=w556:dbl)
      n428 = Multiply(x=w634, y=w622) -> (x*y=w633:dbl)
      n429 = Multiply(x=w694, y=w622) -> (x*y=w693:dbl)
      n430 = Multiply(x=w496, y=w476) -> (x*y=w495:dbl)
      n431 = Multiply(x=w556, y=w476) -> (x*y=w555:dbl)
      n432 = Subtract(x=w635, y=w633) -> (x-y=w625:dbl)
      n433 = Subtract(x=w695, y=w693) -> (x-y=w626:dbl)
      n434 = Subtract(x=w497, y=w495) -> (x-y=w488:dbl)
      n435 = Subtract(x=w557, y=w555) -> (x-y=w489:dbl)
      n436 = case shown="False" w629 {
        tunnel: [w760 w766] -> w628
        tunnel: w622 -> [_ w767]
        tunnel: w627 -> [w763 _]
        tunnel: w626 -> [w762 _]
        tunnel: w625 -> [w761 _]
        frame False {
          n437 = case shown="False" w763 {
            tunnel: [w764 w765] -> w760
            tunnel: w762 -> [_ w765]
            tunnel: w761 -> [w764 _]
            frame False {
            }
            frame True {
            }
          }
        }
        frame True {
          n438 = Subtract(x=1.0, y=w767) -> (x-y=w766:dbl)
        }
      }
      n439 = case shown="False" w491 {
        tunnel: [w751 w757] -> w473
        tunnel: w476 -> [_ w758]
        tunnel: w490 -> [w754 _]
        tunnel: w489 -> [w753 _]
        tunnel: w488 -> [w752 _]
        frame False {
          n440 = case shown="False" w754 {
            tunnel: [w755 w756] -> w751
            tunnel: w753 -> [_ w756]
            tunnel: w752 -> [w755 _]
            frame False {
            }
            frame True {
            }
          }
        }
        frame True {
          n441 = Subtract(x=1.0, y=w758) -> (x-y=w757:dbl)
        }
      }
      n442 = Multiply(x=w628, y=w614) -> (x*y=w613:dbl)
      n443 = Multiply(x=w473, y=w472) -> (x*y=w474:dbl)
    }
    n444 = case shown="True" w96 {
      tunnel: w117 -> [_ w466]
      tunnel: w106 -> [w462 w465]
      tunnel: w116 -> [_ w464]
      tunnel: [w462 w464] -> w97
      tunnel: [w461 w463] -> w84
      tunnel: w90 -> [w461 _]
      frame False {
      }
      frame True {
        n445 = Subtract(x=w466, y=w465) -> (x-y=w463:dbl[])
      }
    }
    n446 = case shown="True" w96 {
      tunnel: w100 -> [_ w460]
      tunnel: w101 -> [w456 w459]
      tunnel: w101 -> [_ w458]
      tunnel: [w456 w458] -> w99
      tunnel: [w455 w457] -> w85
      tunnel: w90 -> [w455 _]
      frame False {
      }
      frame True {
        n447 = Subtract(x=w460, y=w459) -> (x-y=w457:dbl[])
      }
    }
    n448 = Subtract(x=w84, y=w85) -> (x-y=w88:dbl[])
    n449 = Add(x=w84, y=w85) -> (x+y=w86:dbl[])
    n450 = call "rhominus.vi"("Array"=w97, "Array 2"=w99) -> ("Array 3"=w93:dbl[])  [unwired: 9 in]
    n451 = call "P.vi"("Array 3"=w99, "Array in"=w97) -> ("Array out"=w95:dbl[])  [unwired: 9 in]
    n452 = call "rhozero.vi"("Array in"=w99) -> ("Array out"=w94:dbl[])  [unwired: 10 in]
    n453 = Divide(x=w86, y=w83) -> (x/y=w82:dbl[])
    n454 = Subtract(x=w95, y=w94) -> (x-y=w80:dbl[])
    n455 = Divide(x=w88, y=w83) -> (x/y=w81:dbl[])
    n456 = Bundle(w60, "Array out"=w95) -> (w72:cluster{dbl[], "Array out":dbl[]})  [unwired: 1 in]
    n457 = Bundle(w60, "Array out"=w94) -> (w70:cluster{dbl[], "Array out":dbl[]})  [unwired: 1 in]
    n458 = Subtract(x=w94, y=w93) -> (x-y=w79:dbl[])
    n459 = Reverse 1D Array(array=w81) -> (reversed array=w91:dbl[])
    n460 = Bundle(w60, "Array 3"=w93) -> (w69:cluster{dbl[], "Array 3":dbl[]})  [unwired: 1 in]
    n461 = Reverse 1D Array(array=w82) -> (reversed array=w92:dbl[])
    n462 = Build Array(w72, w70, w69) -> (→"Population Graphs":cluster{dbl[], "Array 3":dbl[]}[])
    n463 = Divide(x=w91, y=w83) -> (x/y=w87:dbl[])
    n464 = Divide(x=w92, y=w83) -> (x/y=w89:dbl[])
    n465 = Add(x=w79, y=w87) -> (x+y=w77:dbl[])
    n466 = Add(x=w80, y=w89) -> (x+y=w78:dbl[])
    n467 = Divide(x=12.0, y=500.0) -> (x/y=w45:dbl)
    n468 = Bundle(w60, w77) -> (w66:cluster{dbl[], dbl[]})  [unwired: 1 in]
    n469 = Bundle(w60, w78) -> (w65:cluster{dbl[], dbl[]})  [unwired: 1 in]
    n470 = Divide(x=12.0, y=500.0) -> (x/y=w51:dbl)
    n471 = Add(x=w77, y=w78) -> (x+y=w14:dbl[])
    n472 = Bundle(w60, w14) -> (w67:cluster{dbl[], dbl[]})  [unwired: 1 in]
    n473 = Build Array(w67, w65, w66) -> (→"Corrected Data (P)":cluster{dbl[], dbl[]}[])
    n474 = Add Array Elements(numeric array=w14) -> (sum=w55:dbl)
    n475 = Multiply(x=w55, y=w51) -> (x*y=w52:dbl)
    n476 = Absolute Value(x=w52) -> (abs(x)=w15:dbl)
    "Reimann\nsum of P" <- w15
    n477 = Subtract(x=w78, y=w77) -> (x-y=w53:dbl[])
    n478 = Bundle(w60, w53) -> (→"Corrected Data (Q)":cluster{dbl[], dbl[]})  [unwired: 1 in]
    n479 = Add Array Elements(numeric array=w53) -> (sum=w54:dbl)
    n480 = Multiply(x=w54, y=w45) -> (x*y=w48:dbl)
    n481 = Absolute Value(x=w48) -> (abs(x)=w32:dbl)
    "Reimann \nsum of Q" <- w32
    n482 = Array To Spreadsheet String(delimiter (Tab)=",", array=w14, 3:"%f") -> (spreadsheet string=w8:string)
    n483 = Bundle(w15, w32) -> (→"Total Polarization (P)":cluster{dbl, dbl})  [unwired: 1 in]
    n484 = Format Into String(format string="%d", initial string="", w13) -> (resulting string=w12:string)  [unwired: 1 in, 1 out]
    n485 = Concatenate Strings(w12, ",", w8) -> (w9:string)
    n486 = Write to Text File(file (use dialog)=w21, text=w9, error in=w20) -> (refnum out=w19:refnum<file>, error out=w18:errorcluster)  [unwired: 1 in, 1 out]
  }
  n487 = Close File(refnum=w2, error in=w1) -> ()  [unwired: 2 out]
